vi "Populate FIFO Names in Engine.vi"(7 "Path to SOM Engine":string="IONode\\Controls\\All Nodes Resources.ctl", 8 "error in":errorcluster, 11 "Path to IO Node":path=path "D:/Documents/Projects/SPIAPI/IOEngineCode/Initialize Node Resources.vi") -> (0 "error out":errorcluster, 3 "Path to IO Node":path=path "D:/Documents/Projects/SPIAPI/IOEngineCode/Initialize Node Resources.vi")   [LabVIEW 2014, in "Initialization and IO Node Scripting.lvlib"]
uses:
  Initialization and IO Node Scripting.lvlib
  <vilib>/Utility/traverseref.llb/TRef TravTarget.ctl
  <vilib>/Utility/traverseref.llb/VI Scripting - Traverse.lvlib
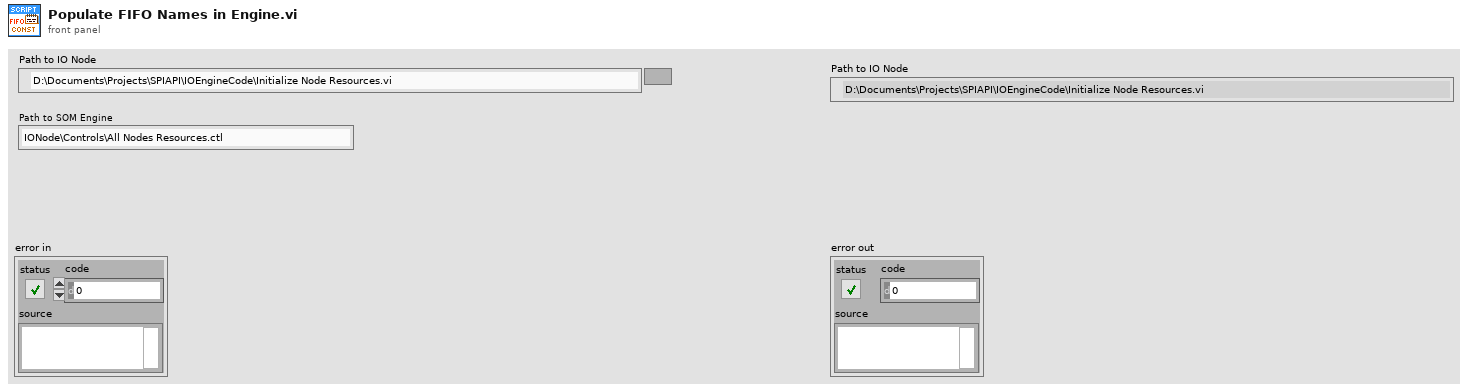
[diagram p1: front panel]
types:
  T1 = typedef "TRef TravTarget.ctl" = enum16{"FP", "BD", "Other"}
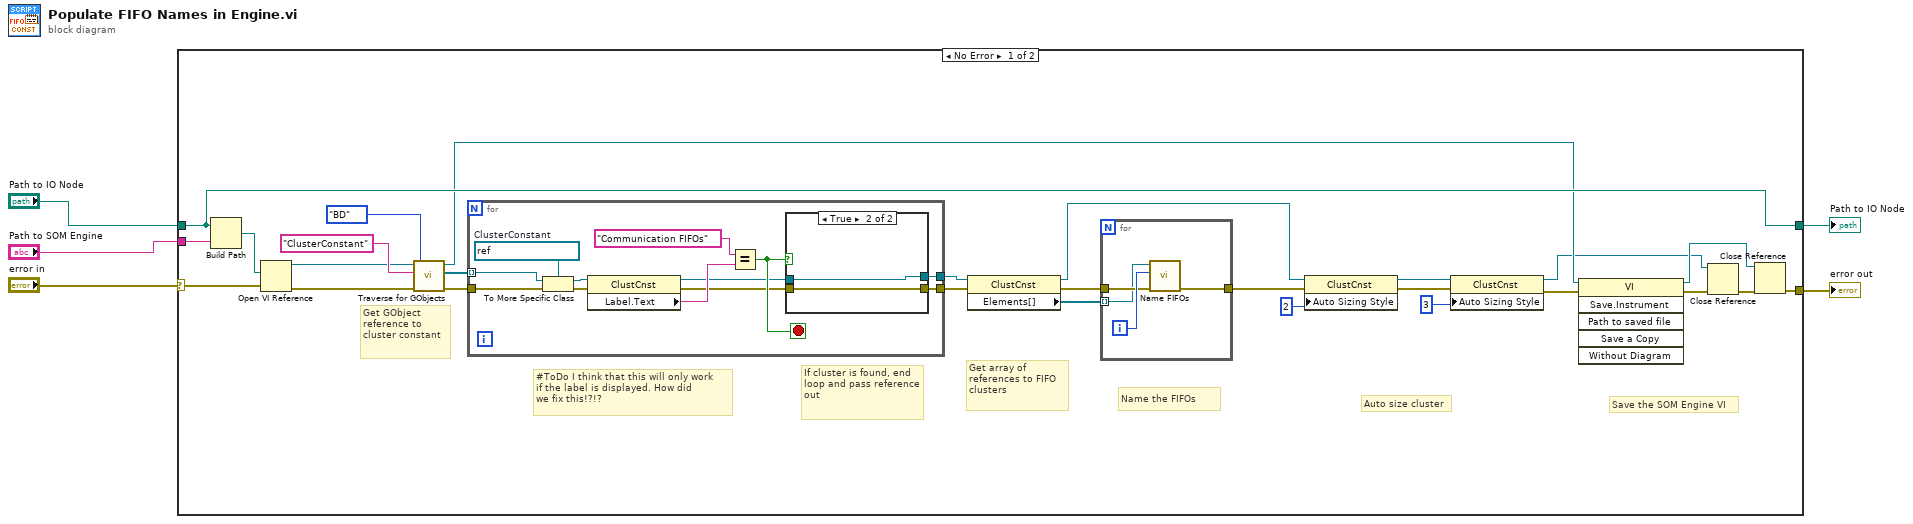
[diagram p0: block diagram]
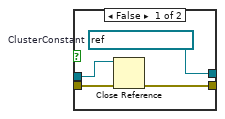
[diagram p2: hidden frame]
diagram:
  n1 = case shown="No Error" "error in" {
    selector: "error in" -> [w31 w56]
    tunnel: [w32 w56] -> w5
    tunnel: "Path to IO Node" -> [w30 w55]
    tunnel: [w30 w55] -> w2
    tunnel: "Path to SOM Engine" -> [w29 _]
    frame No Error {
      # "Save the SOM Engine VI"
      # "Auto size cluster"
      # "Name the FIFOs"
      # "#ToDo I think that this will only work\nif the label is displayed. How did\nwe fix this!?!?"
      # "If cluster is found, end loop and pass reference out"
      # "Get array of references to FIFO clusters"
      # "Get GObject reference to cluster constant"
      n2 = Build Path(base path=w30, name or relative path=w29) -> (appended path=w27:path)
      n3 = Open VI Reference(vi path=w27, error in (no error)=w31) -> (vi reference=w24:refnum<vi>, error out=w23:errorcluster)  [unwired: 4 in]
      n4 = call <vilib>:"Traverse for GObjects.vi"("Traverse Target"=TRef_TravTarget."BD", "error in (no error)"=w23, "Class Name"="ClusterConstant", "VI Refnum"=w24) -> ("error out"=w13:errorcluster, "References"=w14:refnum<vi>[], "dup VI Refnum"=w22:refnum<vi>)  [unwired: 4 in, 1 out]
      n5 = for {
        tunnel: w14 -> [w42] mode=indexing
        tunnel: w13 -> [w43]
        tunnel: [w34] -> w10
        tunnel: [w33] -> w9
        stop <- w37 stop-if-true
        w44 = refnum<vi> refnum  # ClusterConstant
        n6 = To More Specific Class(target class=w44, reference=w42, error in=w43) -> (specific class reference=w40:refnum<vi>, error out=w41:errorcluster)
        n7 = property class="ClustCnst"(reference=w40, error in=w41) -> (reference out=w35:refnum<vi>, error out=w36:errorcluster, "Label.Text"=w39:string)
        n8 = Equal?(x="Communication FIFOs", y=w39) -> (x = y?=w37:bool)
        n9 = case shown="True" w37 {
          tunnel: w36 -> [w48 w50]
          tunnel: w35 -> [w47 w49]
          tunnel: [w45 w50] -> w33
          tunnel: [w46 w49] -> w34
          frame False {
            w46 = refnum<vi> refnum  # ClusterConstant
            n10 = Close Reference(reference=w47, error in (no error)=w48) -> (error out=w45:errorcluster)
          }
          frame True {
          }
        }
      }
      n11 = property class="ClustCnst"(reference=w10, error in=w9) -> (reference out=w6:refnum<vi>, error out=w8:errorcluster, "Elements[]"=w7:refnum<vi>[])
      n12 = for {
        tunnel: [w53] -> w12
        tunnel: w8 -> [w52]
        tunnel: w7 -> [w51] mode=indexing
        i -> [w54]
        n13 = call "Name FIFOs.vi"("error in (no error)"=w52, "Values for Naming"=w54, "Communications FIFOs Element"=w51) -> ("error out"=w53:errorcluster)  [unwired: 8 in]
      }
      n14 = property class="ClustCnst"(reference=w6, error in=w12, "Auto Sizing Style"=u32 2 ("Auto Sizing")) -> (reference out=w19:refnum<vi>, error out=w18:errorcluster)
      n15 = property class="ClustCnst"(reference=w19, error in=w18, "Auto Sizing Style"=u32 3 ("Auto Sizing")) -> (reference out=w15:refnum<vi>, error out=w16:errorcluster)
      n16 = invoke class="VI" method="Save.Instrument"(reference=w22, error in=w16) -> (reference out=w28:refnum<vi>, error out=w11:errorcluster)  [unwired: 4 in, 4 out]
      n17 = Close Reference(reference=w15, error in (no error)=w11) -> (error out=w21:errorcluster)
      n18 = Close Reference(reference=w28, error in (no error)=w21) -> (error out=w32:errorcluster)
    }
    frame Error {
    }
  }
  "error out" <- w5
  "Path to IO Node" <- w2
